vi "PeltierPID_FinalDesign.vi"() -> ()   [LabVIEW 2019]
uses:
  <vilib>/Utility/error.llb/DialogType.ctl
  <vilib>/DAQmx/write.llb/DAQmx Write (Digital Bool 1Line 1Point).vi
  <vilib>/DAQmx/read.llb/DAQmx Read (Analog DBL 1Chan 1Samp).vi
  <vilib>/Analysis/baseanly.llb/Mean (DBL).vi
  <vilib>/DAQmx/create/channels.llb/DAQmx Create Channel (DO-Digital Output).vi
  <vilib>/DAQmx/miscellaneous.llb/DAQmx Fill In Error Info.vi
  PeltierPID_FinalDesignFeb2022/Global 9.vi
  <instrlib>/BK Precision 178XB Series/BK Precision 178XB Series.lvlib
  <vilib>/Analysis/NI_AALBase.lvlib
panel:
  out "averageTemperature":dbl[](array[numeric])
  in  "Integral Allowed?":bool
  out "Integrated error":dbl
  out "Rude Temp":dbl format="%0.2f"
  in  "file (use dialog)":path
  out "error out":errorcluster
  out "Output Voltage":dbl
  in  "dt ( -1 is default)":dbl=-1.0 format="%.3f"
  in  "PID Gain Values":T1={"proportional gain (Kc)"=8.0, "integral time (Ti, min)"=0.1, "derivative time (Td, min)"=0.05} {"derivative time (Td, min)" format="%.3f"; "integral time (Ti, min)" format="%.3f"; "proportional gain (Kc)" format="%.3f"}
  in  "setpoint":dbl format="%.2f"
  out "temp. Graph":dbl(graph)
  out "Output voltage Graph":dbl(graph)
  in  "?":bool
  out "Real-time voltage":dbl format="%.2f"
  out "Thermocouple":dbl
  in  "Current Limit (3 A)":dbl min=0.0 max=6.0 format="%#.2g"
  in  "Maximum Output Voltage (18)":dbl=18.0 min=0.0 max=72.0 format="%#.2f"
  in  "VISA resource name":refnum<visa-resource-name>
  out "Polarity Boolean":bool
  out "Value Change Case structure":bool
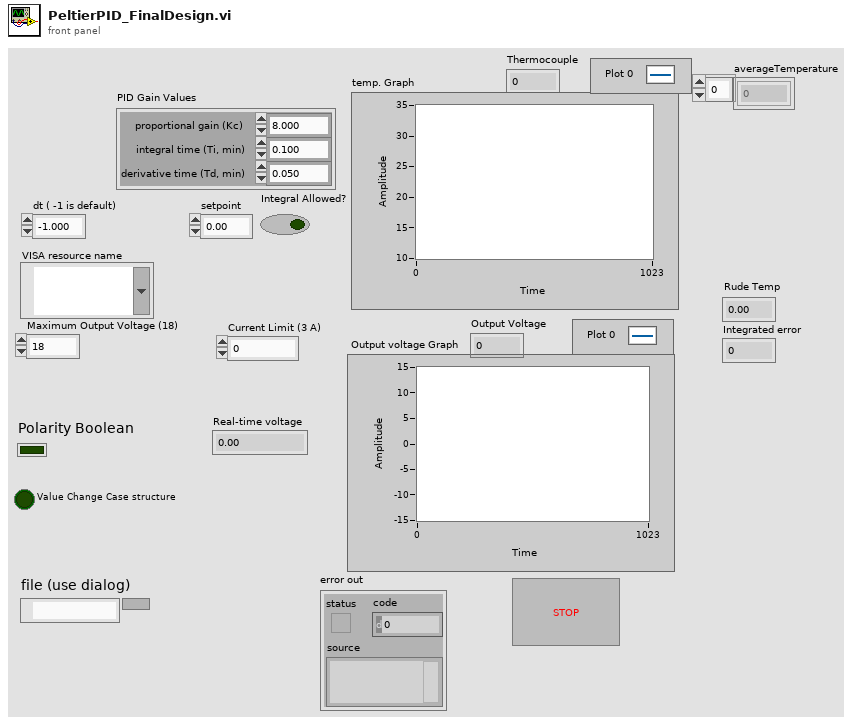
[diagram p1: front panel]
types:
  T1 = cluster{"proportional gain (Kc)":dbl, "integral time (Ti, min)":dbl, "derivative time (Td, min)":dbl}
  T2 = typedef "DialogType.ctl" = u16
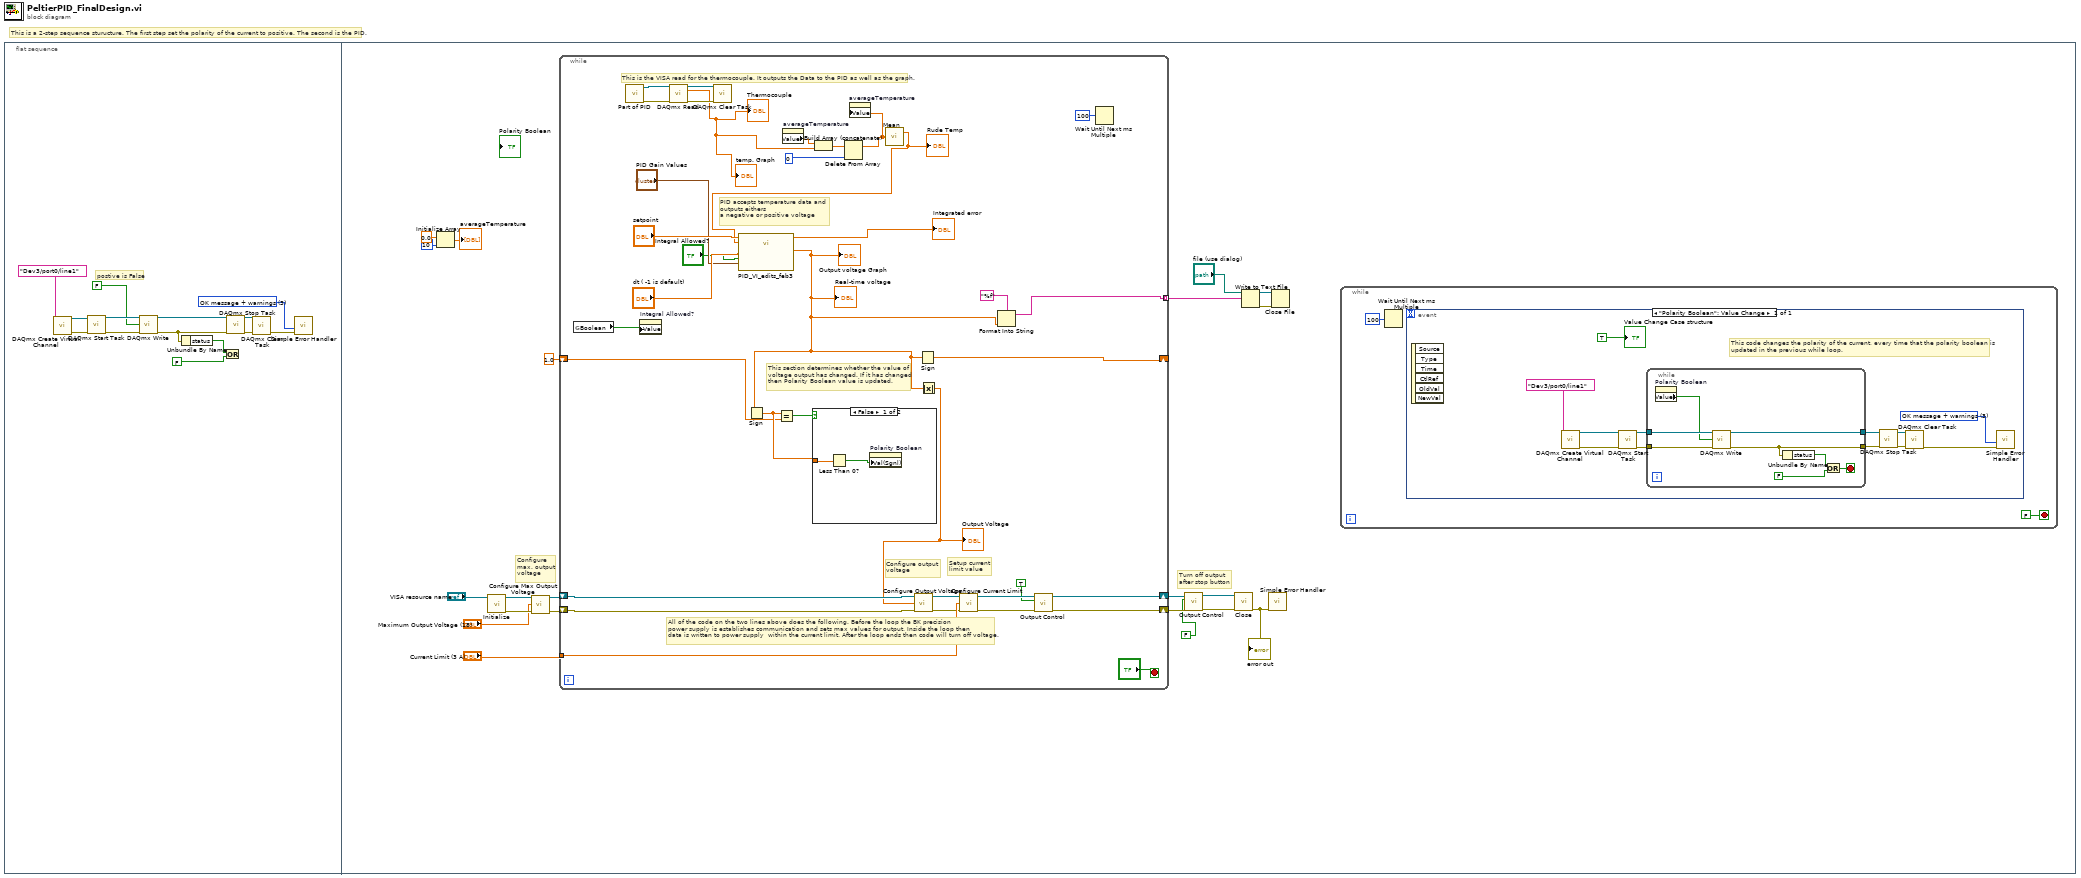
[diagram p0: block diagram]
diagram:
  # "This is a 2-step sequence sturucture. The first step set the polarity of the current to positive. The second is the PID."
  n1 = flat-sequence {
    frame #0 {
      w14 = T2 3 items=["no dialog", "OK message", "continue or stop message", "OK message + warnings", "continue/stop + warnings"] ("type of dialog (OK msg:1)")
      # "postive is False"
      n2 = call-poly <vilib>:"DAQmx Create Virtual Channel.vi"("lines"=tag "Dev3/port0/line1" ("Line(s)")) -> ("task out"=w9:refnum<k21>, "error out"=w8:errorcluster)  [unwired: 13 in]
      n3 = call <vilib>:"DAQmx Start Task.vi"("task/channels in"=w9, "error in"=w8) -> ("task out"=w4:refnum<k21>, "error out"=w5:errorcluster)  [unwired: 12 in]
      n4 = call-poly <vilib>:"DAQmx Write.vi"("task/channels in"=w4, "data"=FALSE ("Reverse Polarity"), "error in"=w5) -> ("task out"=w12:refnum<k21>, "error out"=w13:errorcluster)  [unwired: 10 in, 1 out]
      n5 = Unbundle By Name(w13) -> ("status"=w3:bool)
      n6 = Or(x=w3, y=FALSE ("Stop")) -> ()  [unwired: 1 out]
      n7 = call <vilib>:"DAQmx Stop Task.vi"("task/channels in"=w12, "error in"=w13) -> ("task out"=w10:refnum<k21>, "error out"=w11:errorcluster)  [unwired: 12 in]
      n8 = call <vilib>:"DAQmx Clear Task.vi"("task in"=w10, "error in"=w11) -> ("error out"=w6:errorcluster)  [unwired: 13 in]
      n9 = call <vilib>:"Simple Error Handler.vi"("type of dialog (OK msg:1)"=w14, "error in (no error)"=w6) -> ()  [unwired: 3 in, 5 out]
    }
    frame #1 {
      # "Turn off output\nafter stop button"
      # "Configure\nmax. output\nvoltage"
      n10 = Initialize Array(0.0 ("element"), 10 ("dimension size")) -> (→"averageTemperature":dbl[])
      n11 = call "Initialize.vi"("VISA resource name"="VISA resource name") -> ("error out"=w28:errorcluster, "VISA resource name out"=w27:refnum<visa-resource-name>)  [unwired: 9 in]
      n12 = call "Configure Max Output Voltage.vi"("VISA resource name"=w27, "Maximum Output Voltage (18)"="Maximum Output Voltage (18)", "error in (no error)"=w28) -> ("VISA resource name out"=w29:refnum<visa-resource-name>, "error out"=w30:errorcluster)  [unwired: 11 in]
      n13 = while {
        tunnel: "Current Limit (3 A)" -> [w93]
        shift-right: [w90] -> w32
        shift-left: w29 -> [w92]
        shift-right: [w89] -> w33
        shift-left: w30 -> [w91]
        shift-right: [w77] -> _
        shift-left: 1.0 -> [w76]
        tunnel: [w71] -> w21 mode=indexing
        stop <- "?" stop-if-true
        # "All of the code on the two lines above does the following. Before the loop the BK precision \npower supply is establishes communication and sets max values for output. Inside the loop then \ndata is written to power supply  within the current limit. After the loop ends then code will turn off voltage."
        # "This section determines whether the value of \nvoltage output has changed. If it has changed \nthen Polarity Boolean value is updated."
        # "PID accepts temperature data and outputs eithers \na negative or positive voltage"
        # "This is the VISA read for the thermocouple. It outputs the Data to the PID as well as the graph."
        # "Setup current\nlimit value"
        # "Configure output\nvoltage"
        n14 = global read "Global 9.vi" "Boolean"() -> (w64:bool)
        n15 = call "Part of PID.vi"() -> ("error out"=w79:errorcluster, "task out"=w80:refnum<k21>)  [unwired: 10 in]
        n16 = property on="Integral Allowed?" class="Bool (strict)"("Value"=w64) -> ()  [unwired: 2 in, 2 out]
        n17 = call-poly <vilib>:"DAQmx Read.vi"("task/channels in"=w80, "error in"=w79) -> ("task out"=w81:refnum<k21>, "data"=w62:dbl, "error out"=w82:errorcluster)  [unwired: 11 in]
        "temp. Graph" <- w62
        "Thermocouple" <- w62
        n18 = call <vilib>:"DAQmx Clear Task.vi"("task in"=w81, "error in"=w82) -> ()  [unwired: 13 in, 1 out]
        n19 = property on="averageTemperature" class="Arr (strict)"() -> ("Value"=w63:dbl[])  [unwired: 2 in, 2 out]
        n20 = Build Array (concatenate)(w63, w62) -> (w61:dbl[])
        n21 = Delete From Array(array=w61, index=0) -> (array with subset deleted=w59:dbl[])  [unwired: 1 in, 1 out]
        n22 = property on="averageTemperature" class="Arr (strict)"("Value"=w59) -> ()  [unwired: 2 in, 2 out]
        n23 = call-poly <vilib>:"Mean.vi"("X"=w59) -> ("mean"=w58:dbl)  [unwired: 1 out]
        "Rude Temp" <- w58
        n24 = call "PID_VI_edits_feb3.vi"("Integral allowed?"="Integral Allowed?", "PID gains"="PID Gain Values", "dt (s)"="dt ( -1 is default)", "process variable"=w58, "setpoint"="setpoint") -> ("output"=w67:dbl, "Integrated error"=→"Integrated error":dbl)  [unwired: 4 in, 1 out]
        "Output voltage Graph" <- w67
        "Real-time voltage" <- w67
        n25 = Sign(1:w67) -> (0:w78:dbl)
        n26 = Equal?(x=w78, y=w76) -> (x = y?=w73:bool)
        n27 = case shown="False" w73 {
          tunnel: w78 -> [w94 _]
          frame False {
            n28 = Less Than 0?(x=w94) -> (x < 0?=w95:bool)
            n29 = property on="Polarity Boolean" class="Bool (strict)"("Val(Sgnl)"=w95) -> ()  [unwired: 2 in, 2 out]
          }
          frame True {
          }
        }
        n30 = Sign(1:w67) -> (0:w77:dbl)
        n31 = Absolute Value(x=w67) -> (abs(x)=w74:dbl)
        "Output Voltage" <- w74
        n32 = call "Configure Output Voltage.vi"("VISA resource name"=w92, "Output Voltage (0)"=w74, "error in (no error)"=w91) -> ("VISA resource name out"=w88:refnum<visa-resource-name>, "error out"=w87:errorcluster)  [unwired: 11 in]
        n33 = call "Configure Current Limit.vi"("VISA resource name"=w88, "Current Limit (0)"=w93, "error in (no error)"=w87) -> ("VISA resource name out"=w86:refnum<visa-resource-name>, "error out"=w85:errorcluster)  [unwired: 11 in]
        n34 = Format Into String(format string="%f", w67) -> (resulting string=w71:string)  [unwired: 2 in, 1 out]
        n35 = call "Output Control.vi"("error in (no error)"=w85, "Enable Output Terminals (F: Off)"=TRUE, "VISA resource name"=w86) -> ("error out"=w89:errorcluster, "VISA resource name out"=w90:refnum<visa-resource-name>)  [unwired: 7 in]
        n36 = Wait Until Next ms Multiple(millisecond multiple=u32 100) -> ()  [unwired: 1 out]
      }
      n37 = call "Output Control.vi"("error in (no error)"=w33, "Enable Output Terminals (F: Off)"=FALSE, "VISA resource name"=w32) -> ("error out"=w35:errorcluster, "VISA resource name out"=w34:refnum<visa-resource-name>)  [unwired: 7 in]
      n38 = call "Close.vi"("error in (no error)"=w35, "VISA resource name"=w34) -> ("error out"=w31:errorcluster)  [unwired: 9 in]
      "error out" <- w31
      n39 = Write to Text File(file (use dialog)="file (use dialog)", text=w21) -> (refnum out=w18:refnum<file>, error out=w19:errorcluster)  [unwired: 2 in, 1 out]
      n40 = call <vilib>:"Simple Error Handler.vi"("error in (no error)"=w31) -> ()  [unwired: 4 in, 5 out]
      n41 = Close File(refnum=w18, error in=w19) -> ()  [unwired: 2 out]
      n42 = while {
        stop <- FALSE stop-if-true
        n43 = Wait Until Next ms Multiple(millisecond multiple=u32 100) -> ()  [unwired: 1 out]
        n44 = event shown="[0] \"Polarity Boolean\": Value Change" {
          selector: _ -> [_]
          dyn-events: _ -> [_]
          timeout: _ -> [_]
          event "Polarity Boolean": Value Change {
            w48 = T2 3 items=["no dialog", "OK message", "continue or stop message", "OK message + warnings", "continue/stop + warnings"] ("type of dialog (OK msg:1)")
            # "This code changes the polarity of the current, every time that the polarity boolean is \nupdated in the previous while loop."
            n45 = event-data() -> ()  [unwired: 1 in, 6 out]
            n46 = call-poly <vilib>:"DAQmx Create Virtual Channel.vi"("lines"=tag "Dev3/port0/line1" ("Line(s)")) -> ("task out"=w43:refnum<k21>, "error out"=w42:errorcluster)  [unwired: 13 in]
            n47 = call <vilib>:"DAQmx Start Task.vi"("task/channels in"=w43, "error in"=w42) -> ("task out"=w38:refnum<k21>, "error out"=w39:errorcluster)  [unwired: 12 in]
            n48 = while {
              tunnel: w38 -> [w57]
              tunnel: w39 -> [w56]
              tunnel: [w53] -> w47
              tunnel: [w54] -> w46
              stop <- w55 stop-if-true
              n49 = property on="Polarity Boolean" class="Bool (strict)"() -> ("Value"=w50:bool)  [unwired: 2 in, 2 out]
              n50 = call-poly <vilib>:"DAQmx Write.vi"("task/channels in"=w57, "data"=w50, "error in"=w56) -> ("task out"=w54:refnum<k21>, "error out"=w53:errorcluster)  [unwired: 10 in, 1 out]
              n51 = Unbundle By Name(w53) -> ("status"=w52:bool)
              n52 = Or(x=w52, y=FALSE ("Stop")) -> (x .or. y?=w55:bool)
            }
            n53 = call <vilib>:"DAQmx Stop Task.vi"("task/channels in"=w46, "error in"=w47) -> ("task out"=w44:refnum<k21>, "error out"=w45:errorcluster)  [unwired: 12 in]
            n54 = call <vilib>:"DAQmx Clear Task.vi"("task in"=w44, "error in"=w45) -> ("error out"=w40:errorcluster)  [unwired: 13 in]
            n55 = call <vilib>:"Simple Error Handler.vi"("type of dialog (OK msg:1)"=w48, "error in (no error)"=w40) -> ()  [unwired: 3 in, 5 out]
            "Value Change Case structure" <- TRUE
          }
        }
      }
    }
  }
